vi "Write bool_setting.vi"(10 "bool_setting":T1, 11 "Sig_DA in":refnum<class "Sig_DA.lvclass">) -> (3 "Sig_DA out":refnum<class "Sig_DA.lvclass">)   [LabVIEW 2019, in "Sig_DA.lvclass"]
uses:
  Sig_DA.lvclass
  TypeDef/bool_setting.ctl
  Sig_DA.lvclass/Sig_DA.ctl
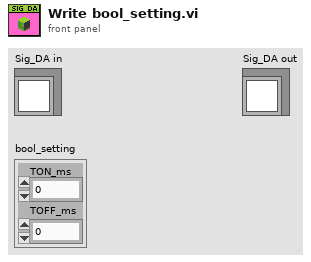
[diagram p1: front panel]
types:
  T1 = typedef "bool_setting.ctl" = cluster{"TON_ms":u32, "TOFF_ms":u32}
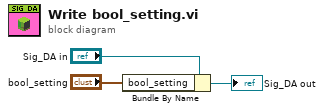
[diagram p0: block diagram]
diagram:
  n1 = Bundle By Name(cluster="Sig_DA in", "bool_setting"="bool_setting") -> (→"Sig_DA out":refnum<class "Sig_DA.lvclass">)
